vi "Find Workspace.vi"(8 "Error In":errorcluster, 9 "Type of Hexaboard":T1, 10 "Control In":T3={"I-O.lvclass"=refnum, "Gantry"=refnum, "Dispenser"="COM1"}, 11 "Workspace In":refnum<class "Pick Up Tool Fixture.lvclass">) -> (0 "Error Out":errorcluster, 1 "Workspace Out":T2, 2 "Control Out":T3={"I-O.lvclass"=refnum, "Gantry"=refnum, "Dispenser"="COM1"}, 3 "Workspace Out":refnum<class "Pick Up Tool Fixture.lvclass">)   [LabVIEW 2021, in "Pick Up Tool Fixture.lvclass"]
uses:
  Pick Up Tool Fixture.lvclass
  C:/Users/hep/Documents/UCSB-CMU-GantryCode/UCSB-Gantry-HEP-main (3)/UCSB-Gantry-HEP-main/Classes/Workspace/Fixture.lvclass
  Controller/Controllers.ctl
  Controller/I-O/I-O.lvclass
  C:/Program Files (x86)/Aerotech/A3200/LabVIEW/2010/Bin/Aerotech.A3200.dll
  Program Files (x86)/Aerotech/A3200/LabVIEW/2010/Bin/Aerotech.A3200.dll
  Workspace.ctl
  Routine/TypeOfHexaboard.ctl
  Fixture.lvclass/Fixture.ctl
  Read Position.vi
  Read Gantry Region.vi
  Fixture.lvclass
  Controller/Controller.lvclass
  Routine/Routine.lvclass
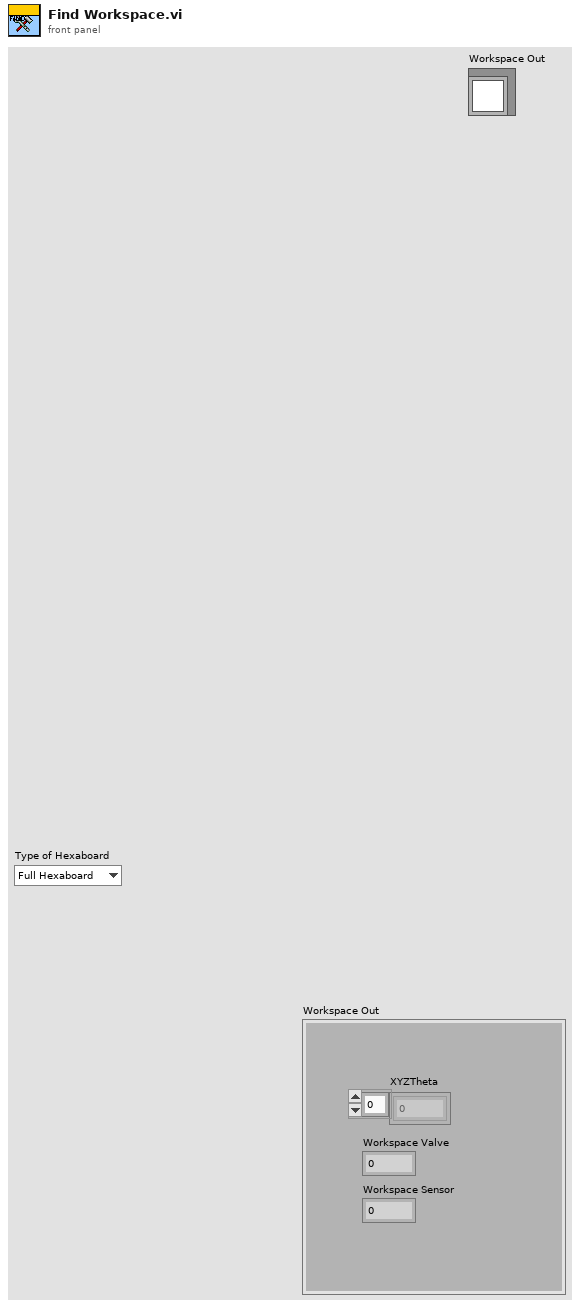
[diagram p1: front panel]
types:
  T1 = typedef "Routine.lvclass/TypeOfHexaboard.ctl" = enum16{"Full Hexaboard", "Right Partial PCB", "Right Partial Sensor", "Al Dummy Right Partial Sensor"}
  T2 = typedef "Fixture.lvclass/Workspace.ctl" = cluster{"XYZTheta":dbl[], "Workspace Valve":i32, "Workspace Sensor":i32}
  T3 = typedef "Controller.lvclass/Controllers.ctl" = cluster{"I-O.lvclass":refnum<class "I-O.lvclass">, "Gantry":refnum<k24>, "Dispenser":refnum<visa-resource-name>}
  T4 = typedef "File Paths.ctl" = cluster{"Glue Pattern Folder":path, "Carrier Tray Folder":path, "Pick Up Tool Fixture Folder":path, "Components Folder":path, "Bellows Tool Offset.txt":path, "Pick Up Tool Offset.txt":path, "Dispense Tip Offset.txt":path, "Log Files":path, "Gantry Assembly Map.txt":path, "Syringe and offset map.txt":path}
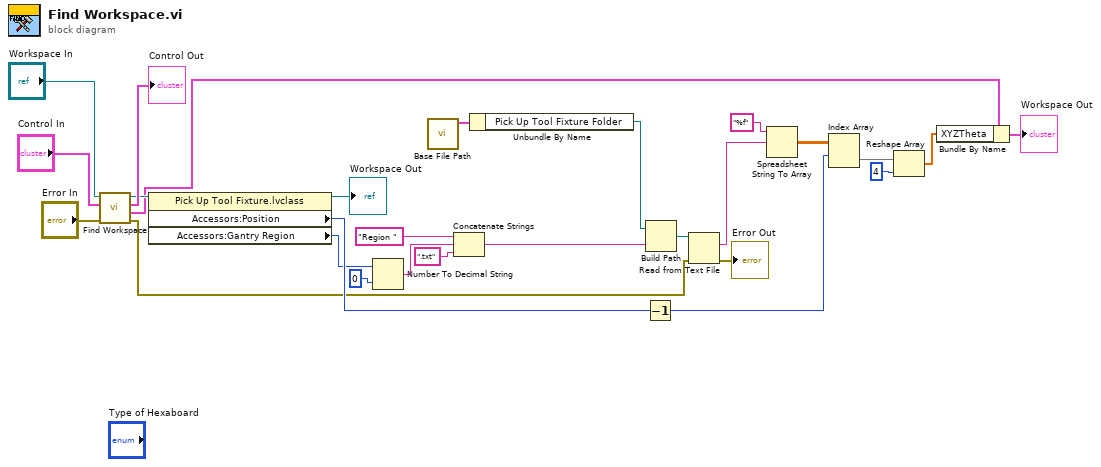
[diagram p0: block diagram]
diagram:
  n1 = call-parent "Find Workspace.vi"("Error In"="Error In", "Control In"="Control In", "Workspace In"="Workspace In") -> ("Error Out"=w2:errorcluster, 1:"Workspace Out"=w10:T2, "Control Out"=→"Control Out":T3, 3:"Workspace Out"=w22:refnum<class "Pick Up Tool Fixture.lvclass">)  [unwired: 5 in]
  n2 = property class="Pick Up Tool Fixture.lvclass"(reference=w22) -> (reference out=→"Workspace Out":refnum<class "Pick Up Tool Fixture.lvclass">, "Accessors:Position"=w6:i32, "Accessors:Gantry Region"=w4:i32)  [unwired: 1 in, 1 out]
  n3 = Number To Decimal String(number=w4, width (-)=i16 0) -> (decimal integer string=w20:string)
  n4 = call "Base File Path.vi"() -> ("Paths Out"=w23:T4)  [unwired: 11 in]
  n5 = Concatenate Strings("Region " ("string"), w20, ".txt") -> (w17:string)
  n6 = Unbundle By Name(w23) -> ("Pick Up Tool Fixture Folder"=w18:path)
  n7 = Decrement(x=w6) -> (x-1=w5:i32)
  n8 = Build Path(base path=w18, name or relative path=w17) -> (appended path=w16:path)
  n9 = Read from Text File(file (use dialog)=w16, error in=w2) -> (text=w15:string, error out=→"Error Out":errorcluster)  [unwired: 2 in, 2 out]
  n10 = Spreadsheet String To Array(format string="%f", spreadsheet string=w15) -> (array=w13:dbl[][])  [unwired: 2 in]
  n11 = Index Array(array=w13, index (row)=w5) -> (element=w12:dbl[])  [unwired: 1 in]
  n12 = Reshape Array(w12, 4 ("dimension size")) -> (w9:dbl[])
  n13 = Bundle By Name(cluster=w10, "XYZTheta"=w9) -> (→"Workspace Out":T2)
